vi "Tree Icons.vi"() -> (1 "Not Selected":i32, 2 "Selected":i32)   [LabVIEW 2021, in "Converter.lvlib"]
uses:
  Converter.lvlib
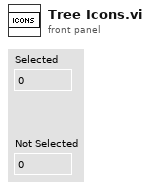
[diagram p1: front panel]
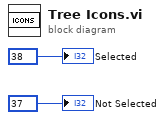
[diagram p0: block diagram]
diagram:
  "Selected" <- 38
  "Not Selected" <- 37
